vi "Audio Filtering (Time Domain).vi"(6 "Filter settings":T1, 8 "error in":errorcluster, 11 "waveforms":waveform(dbl)[](array[waveform])) -> (0 "error out":errorcluster, 3 "time domain":waveform(dbl)[](array[waveform]))   [LabVIEW 2021]
uses:
  <vilib>/addons/_NISVFA/_Shared subVIs/Controls/svc_Window.ctl
  <vilib>/addons/Sound and Vibration/svt_Level/SVL AC & DC Level (Time) (N Ch).vi
  <vilib>/addons/Sound and Vibration/svt_Level/SVL AC & DC Level (Time) (1 Ch).vi
  <vilib>/addons/_NISVFA/_Shared subVIs/Common/svc_Get SV Channel Info.vi
  <vilib>/Analysis/baseanly.llb/Mean.vi
  <vilib>/Analysis/baseanly.llb/Mean (DBL).vi
  <vilib>/addons/_NISVFA/_Shared subVIs/Windowing/svfa_Scaled Time Domain Window (Array).vi
  <vilib>/addons/_NISVFA/_Shared subVIs/Common/svc_Unit Label to Engineering Units.vi
  <vilib>/addons/_NISVFA/_Shared subVIs/Common/svc_Engineering Units to Unit Label.vi
  <vilib>/addons/_NISVFA/_Spectrum Processing/subVIs/svfa_Spectrum Info Window to windowTd Type Def.vi
  <vilib>/Analysis/4window.llb/Force Window.vi
  <vilib>/Analysis/4window.llb/Force Window (DBL).vi
  <vilib>/Analysis/4window.llb/Exponential Window.vi
  <vilib>/Analysis/4window.llb/Exponential Window (DBL).vi
  <vilib>/addons/_NISVFA/_Shared subVIs/Common/svc_Get Window Info.vi
  <vilib>/Analysis/0measdsp.llb/Scaled Time Domain Window.vi
  <vilib>/Analysis/0measdsp.llb/Scaled Time Domain Window (DBL).vi
  <vilib>/Utility/error.llb/Error Cluster From Error Code.vi
  <vilib>/Analysis/baseanly.llb/Std Deviation and Variance.vi
  <vilib>/addons/_NISVFA/_Shared subVIs/Common/svc_Caller VI Returned in Error Source.vi
  <vilib>/addons/Sound and Vibration/svt_Weighting/SVT Audio Filter (N Ch).vi
  <vilib>/addons/Sound and Vibration/svt_Weighting/SVT Weighting Filter (N Ch).vi
  <vilib>/addons/Sound and Vibration/svt_Weighting/SoundVib_ABCWeighting.lvlib
  <vilib>/addons/Sound and Vibration/svt_Weighting/SoundVib_AudioFilter.lvlib
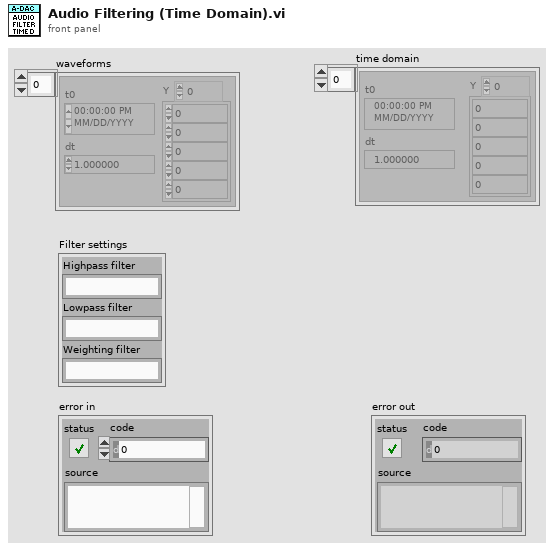
[diagram p1: front panel]
types:
  T1 = cluster{"Highpass filter":string, "Lowpass filter":string, "Weighting filter":string}
  T2 = typedef "svc_Window.ctl" = u32
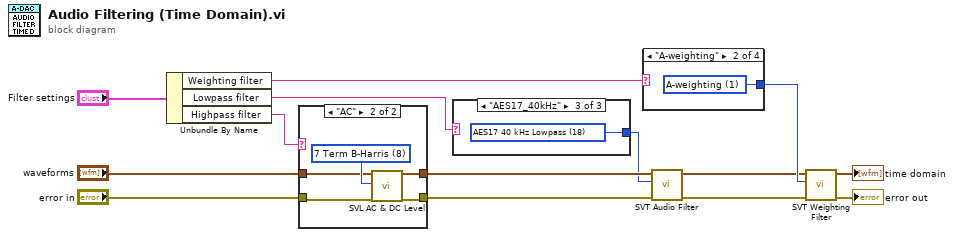
[diagram p0: block diagram]
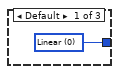
[diagram p2: hidden frame]
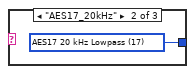
[diagram p3: hidden frame]
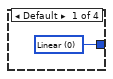
[diagram p4: hidden frame]
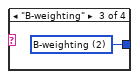
[diagram p5: hidden frame]
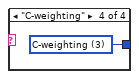
[diagram p6: hidden frame]
diagram:
  n1 = Unbundle By Name("Filter settings") -> ("Weighting filter"=w6:string, "Lowpass filter"=w1:string, "Highpass filter"=w8:string)
  n2 = case shown="\"AC\"" w8 {
    tunnel: "error in" -> [w15 w19]
    tunnel: "waveforms" -> [w16 w20]
    tunnel: [w16 w18] -> w12
    tunnel: [w15 w17] -> w11
    frame "DC", Default {
    }
    frame "AC" {
      w21 = T2 8 items=["None"=0, "Hanning"=1, "Hamming"=2, "Blackman-Harris"=3, "Exact Blackman"=4, "Blackman"=5, "Flat Top"=6, "4 Term B-Harris "=7, "7 Term B-Harris"=8, "Low Sidelobe"=9, "Force"=64, "Exponential"=65, "Blackman Nuttall"=11, "Triangle"=30, "Bartlett-Hanning"=31, "Bohman"=32, "Parzen"=33, "Welch"=34, "Kaiser"=60, "Dolph-Chebyshev"=61, "Gaussian"=62] ("window")
      n3 = call-poly <vilib>:"SVL AC & DC Level.vi"("scaled signals in [EU]"=w20, "window"=w21, "error in (no error)"=w19) -> ("AC signals [EU]"=w18:waveform(dbl)[], "error out"=w17:errorcluster)  [unwired: 11 in, 4 out]
    }
  }
  n4 = case shown="\"AES17_40kHz\"" w1 {
    tunnel: [w22 w23 w24] -> w2
    frame Default {
      w22 = u16 0 items=["Linear"=0, "AES17 20 kHz Lowpass"=17, "AES17 40 kHz Lowpass"=18, "AES17 20 kHz Highpass"=19, "AES17 40 kHz Highpass"=20] ("filter type")
    }
    frame "AES17_20kHz" {
      w23 = u16 17 items=["Linear"=0, "AES17 20 kHz Lowpass"=17, "AES17 40 kHz Lowpass"=18, "AES17 20 kHz Highpass"=19, "AES17 40 kHz Highpass"=20] ("filter type")
    }
    frame "AES17_40kHz" {
      w24 = u16 18 items=["Linear"=0, "AES17 20 kHz Lowpass"=17, "AES17 40 kHz Lowpass"=18, "AES17 20 kHz Highpass"=19, "AES17 40 kHz Highpass"=20] ("filter type")
    }
  }
  n5 = case shown="\"A-weighting\"" w6 {
    tunnel: [w25 w26 w27 w28] -> w5
    frame Default {
      w25 = u16 0 items=["Linear", "A-weighting", "B-weighting", "C-weighting"] ("weighting")
    }
    frame "A-weighting" {
      w26 = u16 1 items=["Linear", "A-weighting", "B-weighting", "C-weighting"] ("weighting")
    }
    frame "B-weighting" {
      w27 = u16 2 items=["Linear", "A-weighting", "B-weighting", "C-weighting"] ("weighting")
    }
    frame "C-weighting" {
      w28 = u16 3 items=["Linear", "A-weighting", "B-weighting", "C-weighting"] ("weighting")
    }
  }
  n6 = call-poly <vilib>:"SVT Audio Filter.vi"("error in (no error)"=w11, "filter type"=w2, "scaled signals [EU]"=w12) -> ("error out"=w3:errorcluster, "filtered signals [EU]"=w4:waveform(dbl)[])  [unwired: 5 in, 2 out]
  n7 = call-poly <vilib>:"SVT Weighting Filter.vi"("error in (no error)"=w3, "weighting"=w5, "scaled signals [EU]"=w4) -> ("error out"=→"error out":errorcluster, "weighted signals [EU]"=→"time domain":waveform(dbl)[])  [unwired: 6 in]
